vi "LOCKOUT.vi"(8 "error in (no error)":errorcluster, 11 "VISA resource name":refnum<visa-resource-name>) -> (0 "error out":errorcluster, 1 "Error Code":i32, 2 "Error Message":string, 3 "VISA resource name out":refnum<visa-resource-name>)   [LabVIEW 2010, in "VITREK V7X.lvlib"]
doc: "Sets the front panel into the <b>REMOTE LOCK-OUT</b> state.\n\n<b>Note:</b> please refer to the instrument manual for the <b>REMOTE LOCK-OUT</b> specification."
uses:
  VITREK V7X.lvlib
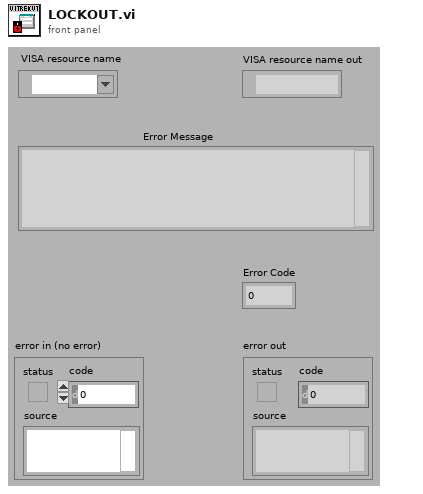
[diagram p1: front panel]
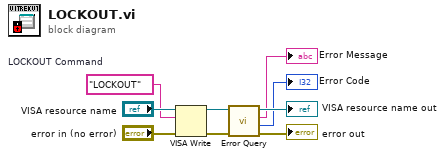
[diagram p0: block diagram]
diagram:
  w7 = "LOCKOUT"  # LOCKOUT Command
  n1 = VISA Write(VISA resource name="VISA resource name", write buffer=w7, error in (no error)="error in (no error)") -> (VISA resource name out=w3:refnum<visa-resource-name>, error out=w4:errorcluster)  [unwired: 1 out]
  n2 = call "Error Query.vi"("error in (no error)"=w4, "VISA resource name"=w3) -> ("error out"=→"error out":errorcluster, "Error Code"=→"Error Code":i32, "Error Message"=→"Error Message":string, "VISA resource name out"=→"VISA resource name out":refnum<visa-resource-name>)  [unwired: 6 in]
